vi "simflight-2.0.vi"() -> ()   [LabVIEW 2014]
uses:
  state space loop data.ctl
  <vilib>/addons/Control Design/_Model Construction/Data Typedefs.llb/CD MIMO Time Response Data.ctl
  <vilib>/addons/Control Design/_Model Construction/Data Typedefs.llb/CD Plot Types Enum.ctl
  <vilib>/Utility/miscctls.llb/LV3DPointTypeDef.ctl
  <vilib>/Analysis/baseanly.llb/Real Outer Product.vi
  Data Xfer/subvis/Curcular Buffer Data History.vi
  <vilib>/Analysis/Matrix/Numeric/Subtract/Subtract - RM,RM.vi
  <vilib>/addons/Control Design/_Model Construction/Model Creation.llb/Model Creation SubVI/cd_Create State Space Model.vi
  <vilib>/Utility/inputDevices.llb/joystickAcquire.vi
  <vilib>/addons/Control Design/_Time Response Analysis/Time Response.llb/Time Response subVI/cd_Linear Simulation (State-Space).vi
  <vilib>/addons/Control Design/_Model Construction/NI_LinSys_Model Creation.lvlib
  <vilib>/addons/Control Design/_Time Response Analysis/NI_CD_Time Response.lvlib
  <vilib>/addons/Control Design/_Model Construction/NI_LinSys_Data Typedefs.lvlib
  attitude indicator/lv-attitudecontrol.lvlib
  <vilib>/Analysis/NI_AALBase.lvlib
  <vilib>/Analysis/Matrix/NI_Matrix.lvlib
panel:
  out "altitude 3":T1(graph)
  out "altitude 2":T1(graph)
  out "altitude":T1(graph)
  in  "elevator gain":dbl
  in  "aileron gain":dbl
  in  "rudder gain":dbl
  out "plot":T1(graph)
  in  "Aircraft":string="MPX5"
  in  "Attitude Indicator":refnum<vi>(3d-picture)
  out "Airspeed (ft/s)":dbl(knob)=74.91519927978516 scale=0.0..120.0 scale format="%#.4f"
  out "motor (BHP)":dbl(slide) scale=-0.2..0.2
  out "ground track":cluster{"Time Stamp":dbl, "Data Value":dbl}[](graph)
  out "roll":dbl(slide) scale=-90.0..90.0
  out "pitch":dbl(slide) scale=-90.0..90.0
  out "rudder":dbl(slide) scale=-25.0..25.0
  out "aileron":dbl(slide) scale=-25.0..25.0
  out "elevator":dbl(slide) scale=-25.0..25.0
  out "Heading":T2(graph)={"X"=[{"Y"=[21.620706805998168, 20.15124367946963, 12.465582235692763, 7.946576972490323, 11.656565240893995, 3.970903792227472, 5.440366929130449, 13.126028372052978, 19.003880895383112, 16.244982298473555, 16.832767550897515, 24.922937499080067, 24.33515224168201, 19.81289788882929, 13.93504536742159, 21.620706805998168], "Y"=[7.099604990531346, 5.077062500919932, 10.661022401488875, 5.291796067500631, 11.248807654089271, 16.832767550897515, 18.855310035128806, 13.271350139939326, 21.36152008350073, 25.220079209877188, 26.02909620777253, 20.151243679469633, 19.34222668734553, 20.773734831883043, 12.683564887248515, 7.099604990531346]}], "z"=[{"Y"=[15.0, 16.30733614, 17.60472267, 17.43107449, 17.60472267, 18.88228568, 20.13030215, 19.78828201, 20.13030215, 21.33927393, 22.5, 22.0, 22.5, 23.60364655, 24.64181415, 23.99902654, 24.64181415, 25.60660172, 26.49066665, 25.7246222, 26.49066665, 27.28728066, 27.99038106, 27.12435565, 27.99038106, 28.59461681, 29.09538931, 28.15569669, 29.09538931, 29.48888739, 29.7721163, 28.78730854, 29.7721163, 29.94292047, 30.0, 28.5, 30.0, 29.94292047, 29.7721163, 28.78730854, 29.7721163, 29.48888739, 29.09538931, 28.15569669, 29.09538931, 28.59461681, 27.99038106, 27.12435565, 27.99038106, 27.28728066, 26.49066665, 25.7246222, 26.49066665, 25.60660172, 24.64181415, 23.99902654, 24.64181415, 23.60364655, 22.5, 22.0, 22.5, 21.33927393, 20.13030215, 19.78828201, 20.13030215, 18.88228568, 17.60472267, 17.43107449, 17.60472267, 16.30733614, 15.0, 15.0, 15.0, 13.69266386, 12.39527733, 12.56892551, 12.39527733, 11.11771432, 9.86969785, 10.21171799, 9.86969785, 8.660726074, 7.5, 8.0, 7.5, 6.396353455, 5.358185855, 6.000973464, 5.358185855, 4.393398282, 3.509333353, 4.275377796, 3.509333353, 2.712719336, 2.009618943, 2.875644347, 2.009618943, 1.405383194, 0.904610688, 1.844303309, 0.904610688, 0.511112606, 0.227883705, 1.212691458, 0.227883705, 0.057079529, 0.0, 1.5, 0.0, 0.057079529, 0.227883705, 1.212691458, 0.227883705, 0.511112606, 0.904610688, 1.844303309, 0.904610688, 1.405383194, 2.009618943, 2.875644347, 2.009618943, 2.712719336, 3.509333353, 4.275377796, 3.509333353, 4.393398282, 5.358185855, 6.000973464, 5.358185855, 6.396353455, 7.5, 8.0, 7.5, 8.660726074, 9.86969785, 10.21171799, 9.86969785, 11.11771432, 12.39527733, 12.56892551, 12.39527733, 13.69266386, 15.0, 15.0], "Y"=[30.0, 29.94292047, 29.7721163, 28.78730854, 29.7721163, 29.48888739, 29.09538931, 28.15569669, 29.09538931, 28.59461681, 27.99038106, 27.12435565, 27.99038106, 27.28728066, 26.49066665, 25.7246222, 26.49066665, 25.60660172, 24.64181415, 23.99902654, 24.64181415, 23.60364655, 22.5, 22.0, 22.5, 21.33927393, 20.13030215, 19.78828201, 20.13030215, 18.88228568, 17.60472267, 17.43107449, 17.60472267, 16.30733614, 15.0, 15.0, 15.0, 13.69266386, 12.39527733, 12.56892551, 12.39527733, 11.11771432, 9.86969785, 10.21171799, 9.86969785, 8.660726074, 7.5, 8.0, 7.5, 6.396353455, 5.358185855, 6.000973464, 5.358185855, 4.393398282, 3.509333353, 4.275377796, 3.509333353, 2.712719336, 2.009618943, 2.875644347, 2.009618943, 1.405383194, 0.904610688, 1.844303309, 0.904610688, 0.511112606, 0.227883705, 1.212691458, 0.227883705, 0.057079529, 0.0, 1.5, 0.0, 0.057079529, 0.227883705, 1.212691458, 0.227883705, 0.511112606, 0.904610688, 1.844303309, 0.904610688, 1.405383194, 2.009618943, 2.875644347, 2.009618943, 2.712719336, 3.509333353, 4.275377796, 3.509333353, 4.393398282, 5.358185855, 6.000973464, 5.358185855, 6.396353455, 7.5, 8.0, 7.5, 8.660726074, 9.86969785, 10.21171799, 9.86969785, 11.11771432, 12.39527733, 12.56892551, 12.39527733, 13.69266386, 15.0, 15.0, 15.0, 16.30733614, 17.60472267, 17.43107449, 17.60472267, 18.88228568, 20.13030215, 19.78828201, 20.13030215, 21.33927393, 22.5, 22.0, 22.5, 23.60364655, 24.64181415, 23.99902654, 24.64181415, 25.60660172, 26.49066665, 25.7246222, 26.49066665, 27.28728066, 27.99038106, 27.12435565, 27.99038106, 28.59461681, 29.09538931, 28.15569669, 29.09538931, 29.48888739, 29.7721163, 28.78730854, 29.7721163, 29.94292047, 30.0, 28.5]}]}
  in  "visual":refnum<k7>(container) caption="3D 파라미터형 표면"
  in  "stop":bool
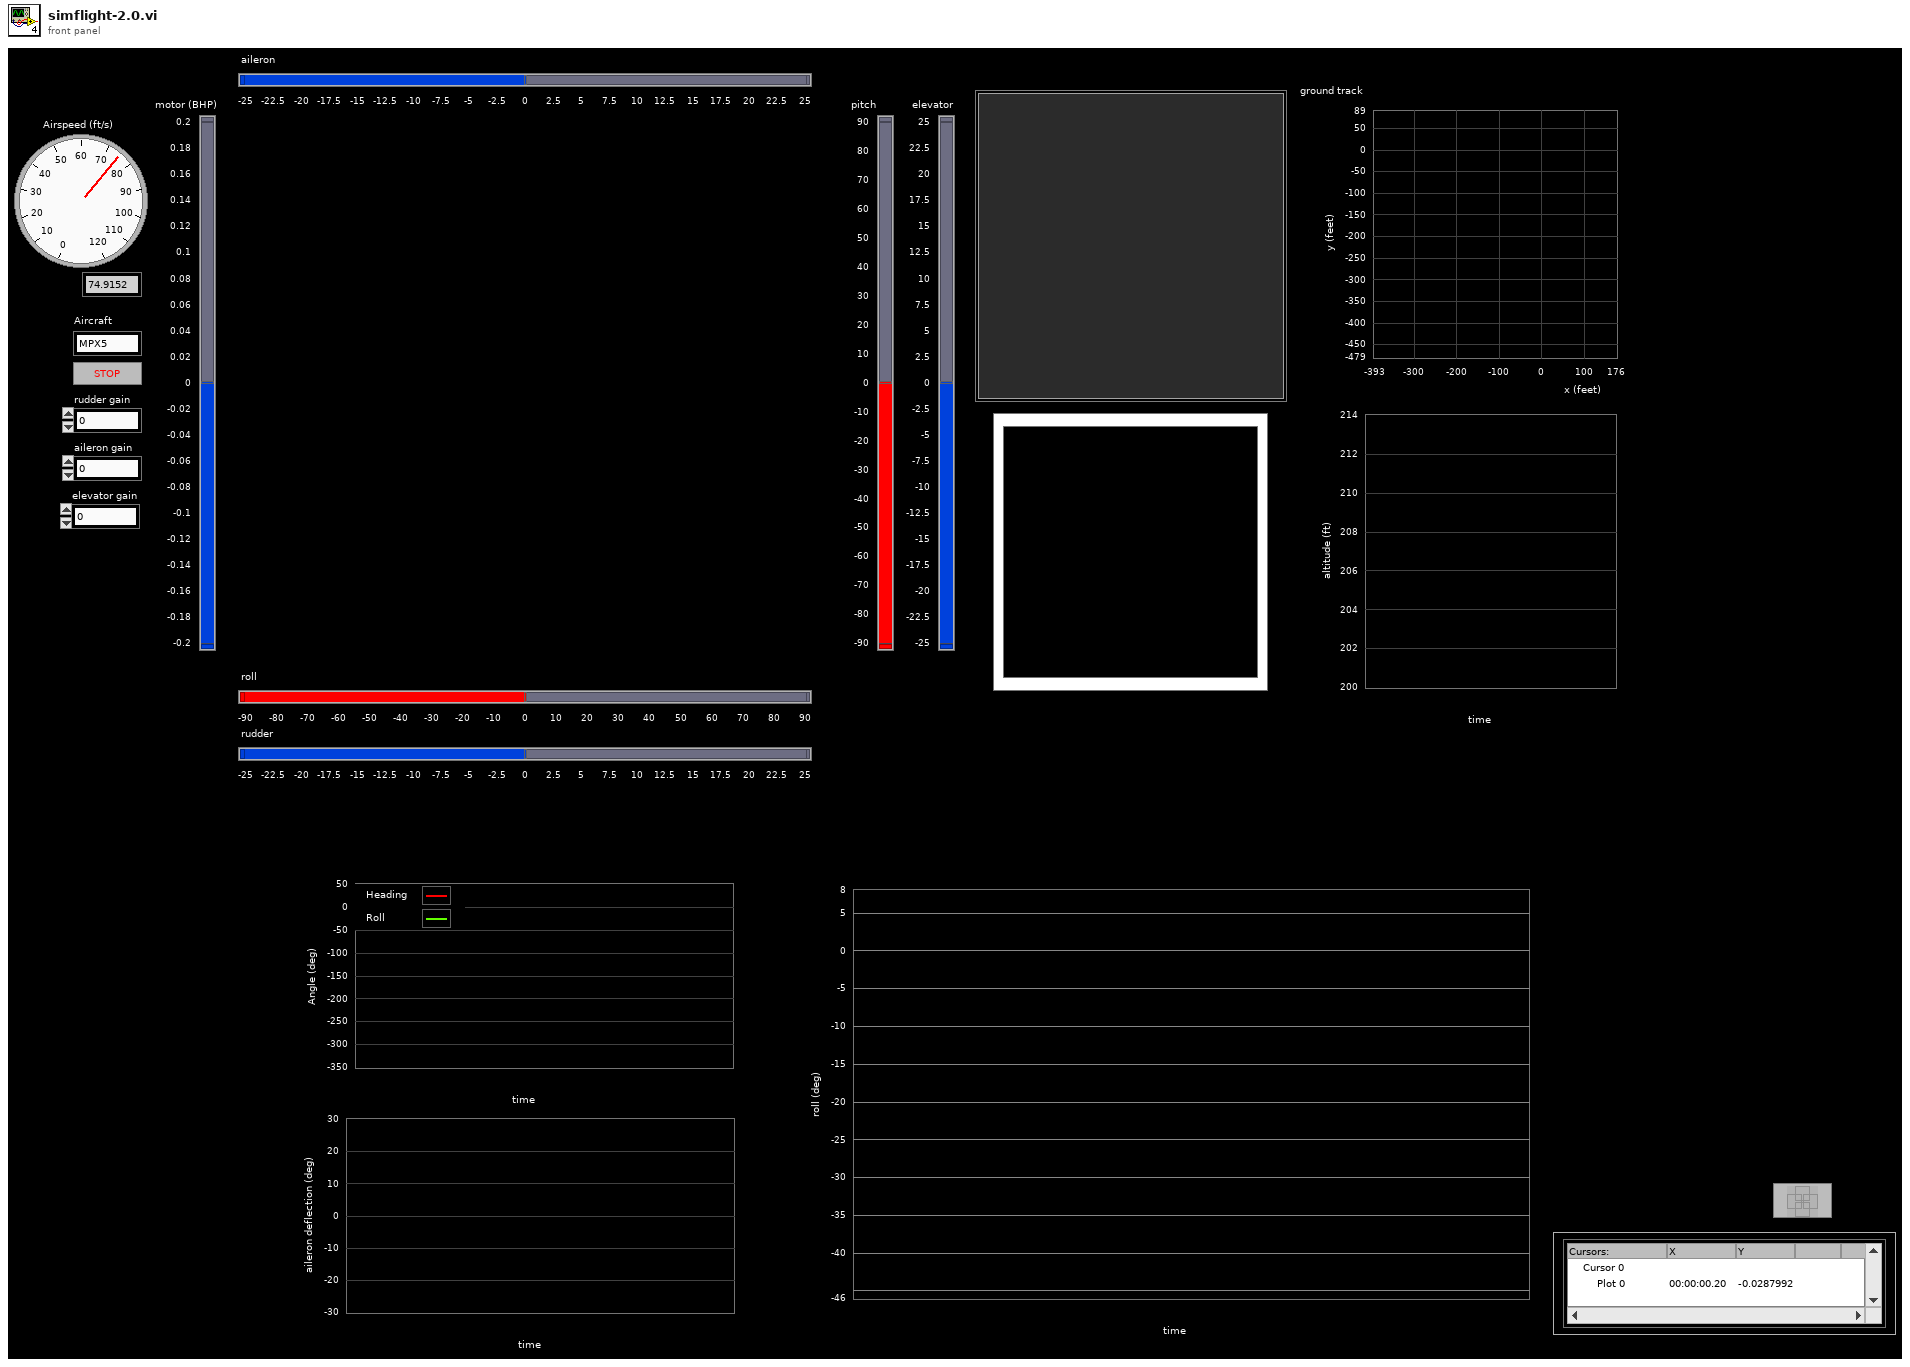
[diagram p1: front panel]
types:
  T1 = cluster{cluster{"Time Stamp":dbl, "Data Value":dbl}[]}[]
  T2 = cluster{"X":cluster{"Y":dbl[], "Y":dbl[]}[], "z":cluster{"Y":dbl[], "Y":dbl[]}[]}
  T3 = typedef "state space loop data.ctl" = cluster{"d_elevator (rad)":dbl, "d_rudder (rad)":dbl, "d_aileron (rad)":dbl, "d_motor (bhp)":dbl, "loop start (s)":dbl, "dT":dbl, "time now":dbl, "Sim Data":T4, "sim conditions":dbl[], "timestamp":dbl}
  T4 = typedef "NI_LinSys_Data Typedefs.lvlib/CD MIMO Time Response Data.ctl" = cluster{"Time":dbl[], "Outputs Data":dbl[][][], "States Data":dbl[][][], "plot type":T5}
  T5 = typedef "NI_LinSys_Data Typedefs.lvlib/CD Plot Types Enum.ctl" = enum16{"bode-magnitude", "bode-phase", "nichols", "nyquist", "singular values", "step", "impulse", "initial", "simulation", "nyquist with separation"}
  T6 = typedef "NI_Matrix.lvlib/RealMatrix.ctl" = dbl[][]
  T7 = typedef "NI_LinSys_Model Typedefs.lvlib/CD State Space Model (MIMO).ctl" = cluster{"properties":T8, "A":dbl[][], "B":dbl[][], "C":dbl[][], "D":dbl[][], "StateNames":string[], "Transport Delay":dbl[][]}
  T8 = typedef "NI_LinSys_Model Typedefs.lvlib/CD General Elements.ctl" = cluster{"Model name":string, "Input names":string[], "Output names":string[], "Input Delays":dbl[], "Output Delays":dbl[], "Sampling Time":dbl, "Notes":string}
  T9 = typedef "lv-attitudecontrol.lvlib/AttitudeHandle.ctl" = cluster{"First Scene Object":refnum<vi>, "Drum":refnum<vi>, "Window":refnum<vi>, "Dial":refnum<vi>, "Scene Graph":refnum<vi>, "Last Drum Pitch":dbl, "Last Drum Roll ":dbl, "Last Dial Roll":dbl}
  T10 = cluster{"X axis":i32, "Y axis":i32, "Z axis":i32, "X axis rotation":i32, "Y axis rotation":i32, "Z axis rotation":i32, "U axis":i32, "V axis":i32}
  T11 = typedef "LV3DPointTypeDef.ctl" = cluster{"X":sgl, "Y":sgl, "Z":sgl}
  T12 = cluster{cluster{"Time Stamp":dbl, "Data Value":dbl}[]}
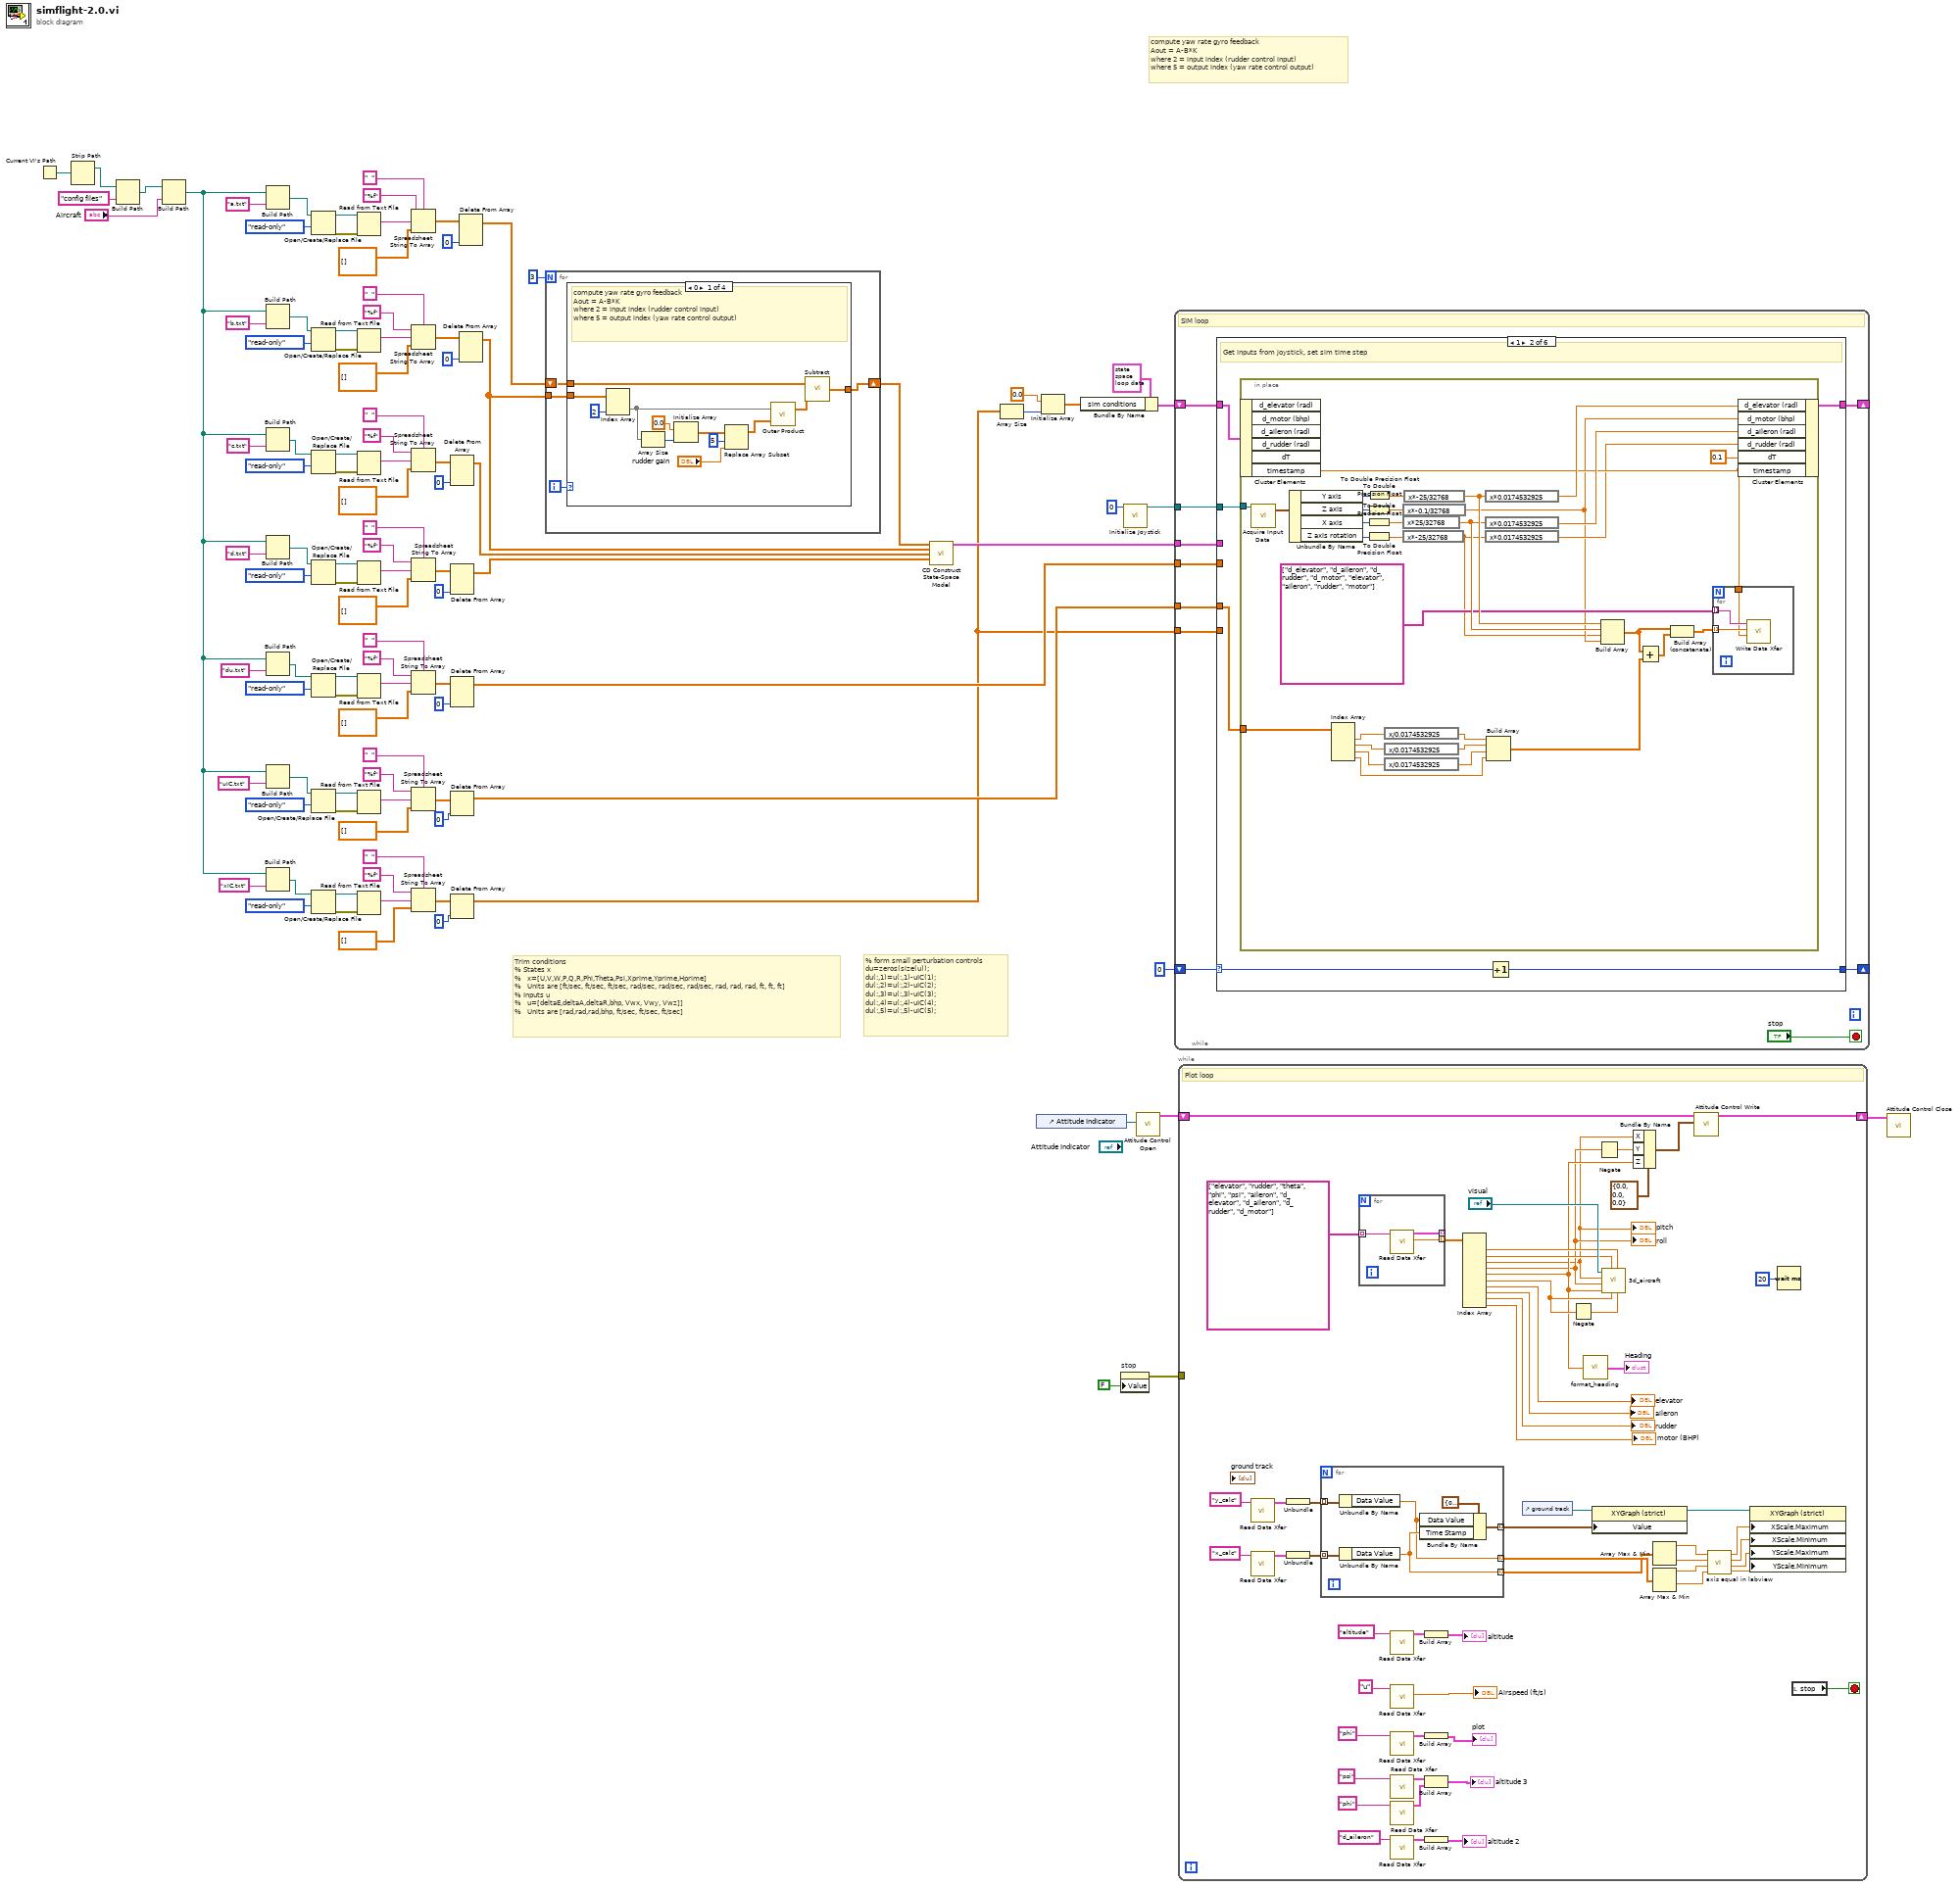
[diagram p0: block diagram]
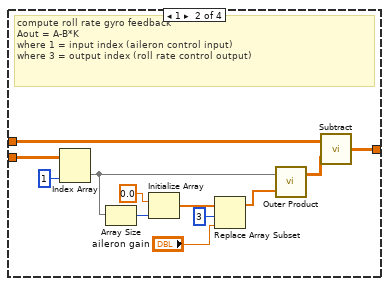
[diagram p2: hidden frame]
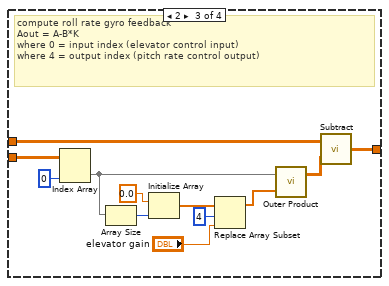
[diagram p3: hidden frame]
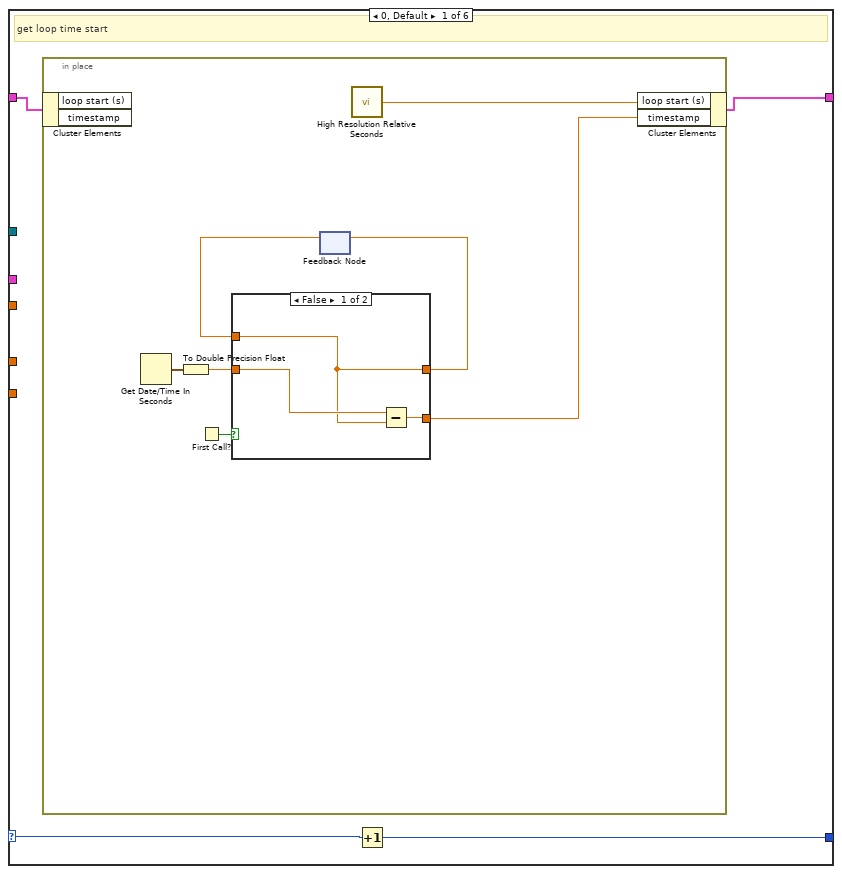
[diagram p5: hidden frame]
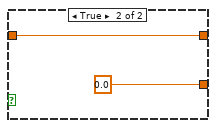
[diagram p6: hidden frame]
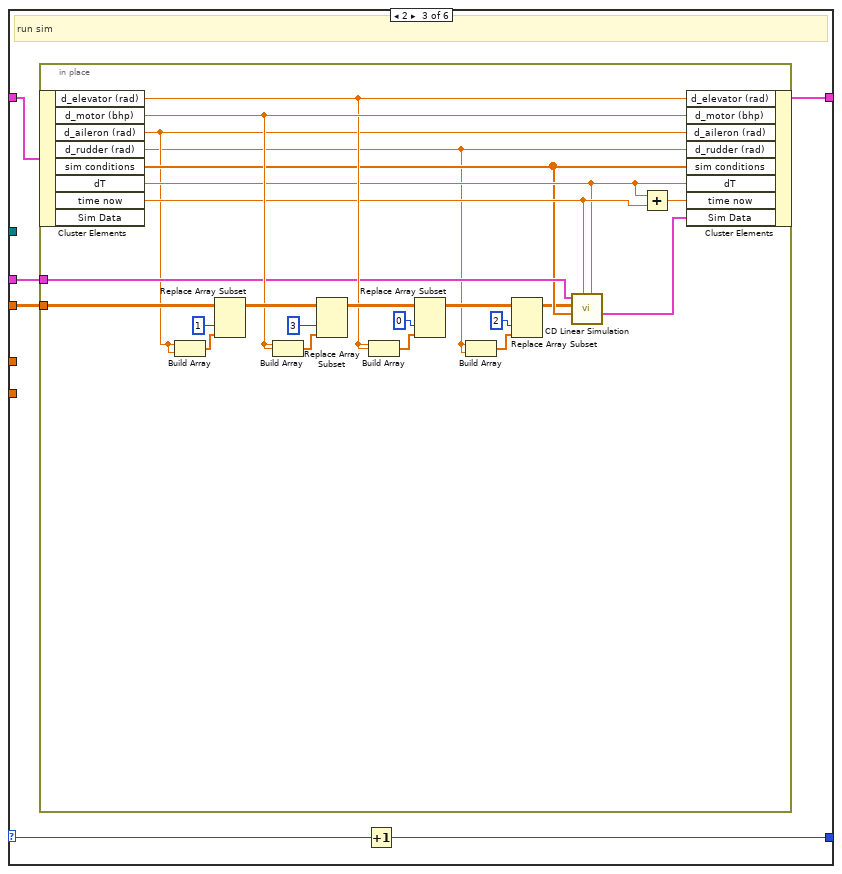
[diagram p7: hidden frame]
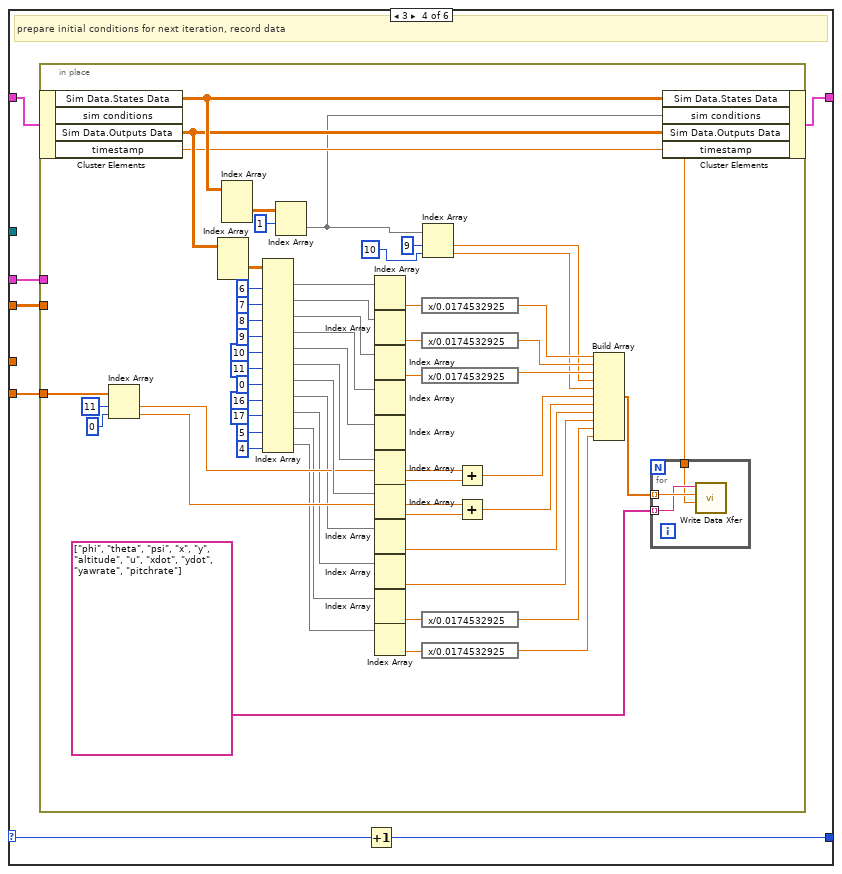
[diagram p8: hidden frame]
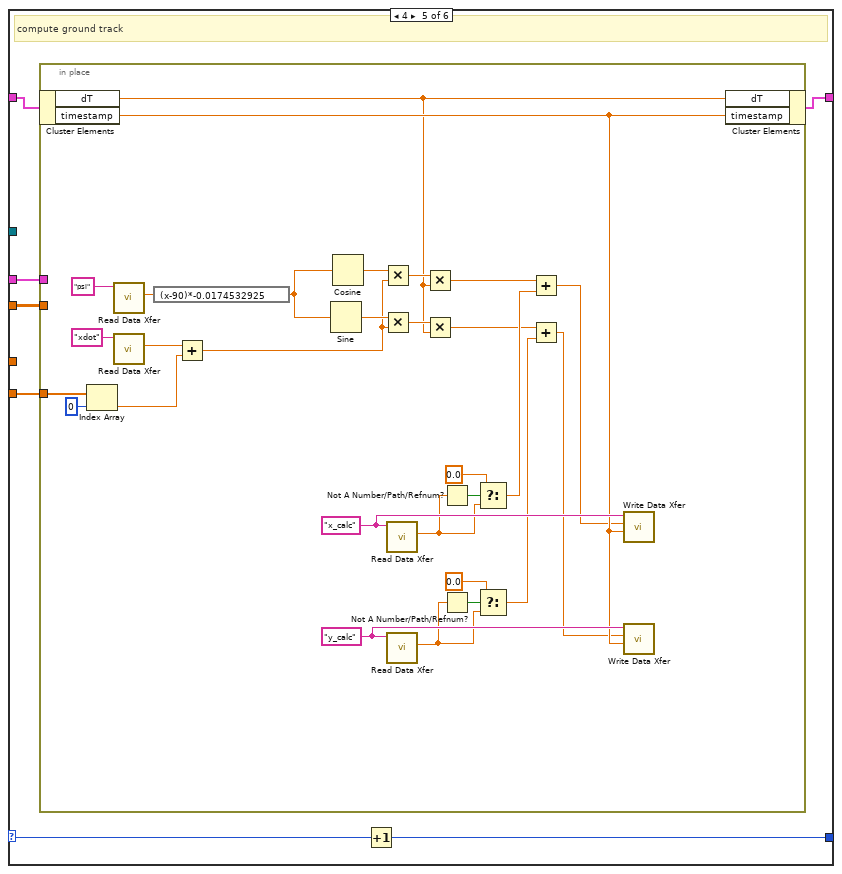
[diagram p9: hidden frame]
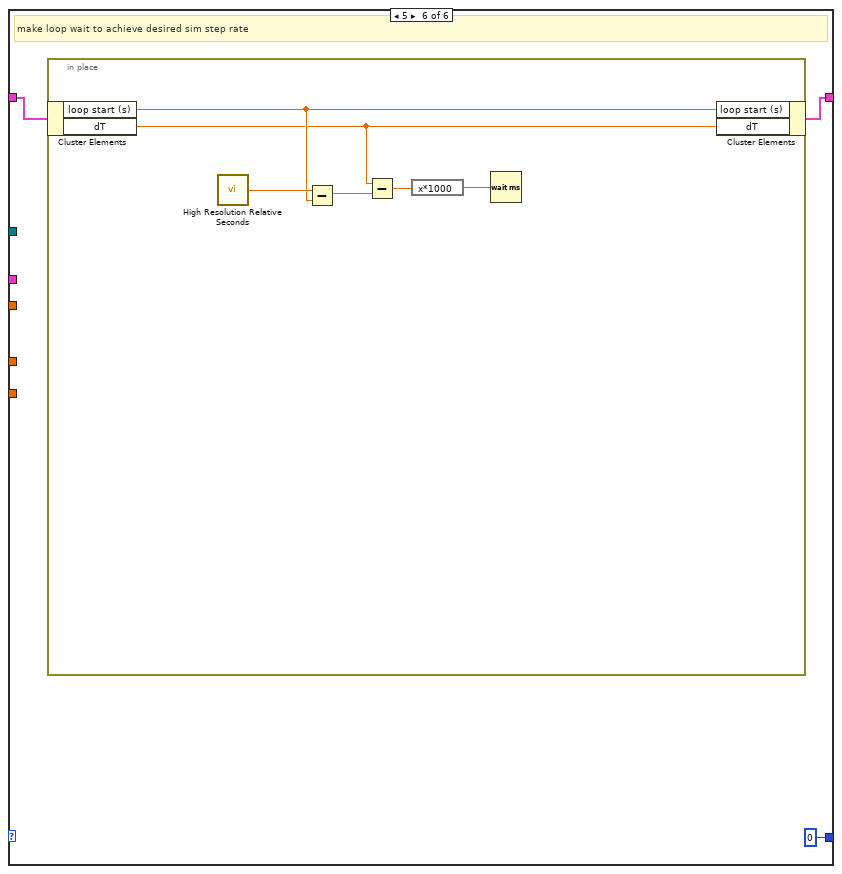
[diagram p10: hidden frame]
diagram:
  # "compute yaw rate gyro feedback\nAout = A-B*K\nwhere 2 = input index (rudder control input)\nwhere 5 = output index (yaw rate control output)"
  # "% form small perturbation controls\ndu=zeros(size(u));\ndu(:,1)=u(:,1)-uIC(1);\ndu(:,2)=u(:,2)-uIC(2);\ndu(:,3)=u(:,3)-uIC(3);\ndu(:,4)=u(:,4)-uIC(4);\ndu(:,5)=u(:,5)-uIC(5);"
  # "Trim conditions\n% States x\n%   x=[U,V,W,P,Q,R,Phi,Theta,Psi,Xprime,Yprime,Hprime]\n%   Units are [ft/sec, ft/sec, ft/sec, rad/sec, rad/sec, rad/sec, rad, rad, rad, ft, ft, ft]\n% Inputs u\n%   u=[deltaE,deltaA,deltaR,bhp, Vwx, Vwy, Vwz]]\n%   Units are [rad,rad,rad,bhp, ft/sec, ft/sec, ft/sec]"
  n1 = Current VI's Path() -> (path=w34:path)
  n2 = Strip Path(path=w34) -> (stripped path=w33:path)  [unwired: 1 out]
  n3 = Build Path(base path=w33, name or relative path="config files") -> (appended path=w50:path)
  n4 = Build Path(base path=w50, name or relative path="Aircraft") -> (appended path=w32:path)
  n5 = Build Path(base path=w32, name or relative path="a.txt") -> (appended path=w47:path)
  n6 = Build Path(base path=w32, name or relative path="b.txt") -> (appended path=w45:path)
  n7 = Build Path(base path=w32, name or relative path="c.txt") -> (appended path=w43:path)
  n8 = Build Path(base path=w32, name or relative path="d.txt") -> (appended path=w41:path)
  n9 = Build Path(base path=w32, name or relative path="du.txt") -> (appended path=w39:path)
  n10 = Build Path(base path=w32, name or relative path="uIC.txt") -> (appended path=w37:path)
  n11 = Build Path(base path=w32, name or relative path="xIC.txt") -> (appended path=w35:path)
  n12 = Open/Create/Replace File(file path (use dialog)=w47, access (0:read/write)=enum16{"read/write", "read-only", "write-only"}."read-only") -> (refnum out=w104:refnum<file>, error out=w105:errorcluster)  [unwired: 4 in, 1 out]
  n13 = Open/Create/Replace File(file path (use dialog)=w45, access (0:read/write)=enum16{"read/write", "read-only", "write-only"}."read-only") -> (refnum out=w97:refnum<file>, error out=w96:errorcluster)  [unwired: 4 in, 1 out]
  n14 = Open/Create/Replace File(file path (use dialog)=w43, access (0:read/write)=enum16{"read/write", "read-only", "write-only"}."read-only") -> (refnum out=w92:refnum<file>, error out=w93:errorcluster)  [unwired: 4 in, 1 out]
  n15 = Open/Create/Replace File(file path (use dialog)=w41, access (0:read/write)=enum16{"read/write", "read-only", "write-only"}."read-only") -> (refnum out=w85:refnum<file>, error out=w84:errorcluster)  [unwired: 4 in, 1 out]
  n16 = Open/Create/Replace File(file path (use dialog)=w39, access (0:read/write)=enum16{"read/write", "read-only", "write-only"}."read-only") -> (refnum out=w80:refnum<file>, error out=w81:errorcluster)  [unwired: 4 in, 1 out]
  n17 = Open/Create/Replace File(file path (use dialog)=w37, access (0:read/write)=enum16{"read/write", "read-only", "write-only"}."read-only") -> (refnum out=w63:refnum<file>, error out=w64:errorcluster)  [unwired: 4 in, 1 out]
  n18 = Open/Create/Replace File(file path (use dialog)=w35, access (0:read/write)=enum16{"read/write", "read-only", "write-only"}."read-only") -> (refnum out=w74:refnum<file>, error out=w75:errorcluster)  [unwired: 4 in, 1 out]
  n19 = Read from Text File(file (use dialog)=w104, error in=w105) -> (text=w103:string)  [unwired: 2 in, 3 out]
  n20 = Read from Text File(file (use dialog)=w97, error in=w96) -> (text=w98:string)  [unwired: 2 in, 3 out]
  n21 = Read from Text File(file (use dialog)=w92, error in=w93) -> (text=w91:string)  [unwired: 2 in, 3 out]
  n22 = Read from Text File(file (use dialog)=w85, error in=w84) -> (text=w86:string)  [unwired: 2 in, 3 out]
  n23 = Read from Text File(file (use dialog)=w80, error in=w81) -> (text=w79:string)  [unwired: 2 in, 3 out]
  n24 = Read from Text File(file (use dialog)=w63, error in=w64) -> (text=w62:string)  [unwired: 2 in, 3 out]
  n25 = Read from Text File(file (use dialog)=w74, error in=w75) -> (text=w73:string)  [unwired: 2 in, 3 out]
  n26 = Spreadsheet String To Array(delimiter (Tab)="  ", format string="%f", spreadsheet string=w103, array type (2D Dbl)=dbl[][] []) -> (array=w20:dbl[][])
  n27 = Spreadsheet String To Array(delimiter (Tab)="  ", format string="%f", spreadsheet string=w98, array type (2D Dbl)=dbl[][] []) -> (array=w17:dbl[][])
  n28 = Spreadsheet String To Array(delimiter (Tab)="  ", format string="%f", spreadsheet string=w91, array type (2D Dbl)=dbl[][] []) -> (array=w14:dbl[][])
  n29 = Spreadsheet String To Array(delimiter (Tab)="  ", format string="%f", spreadsheet string=w86, array type (2D Dbl)=dbl[][] []) -> (array=w11:dbl[][])
  n30 = Spreadsheet String To Array(delimiter (Tab)="  ", format string="%f", spreadsheet string=w79, array type (2D Dbl)=dbl[][] []) -> (array=w8:dbl[][])
  n31 = Spreadsheet String To Array(delimiter (Tab)="  ", format string="%f", spreadsheet string=w62, array type (2D Dbl)=dbl[] []) -> (array=w6:dbl[])
  n32 = Spreadsheet String To Array(delimiter (Tab)="  ", format string="%f", spreadsheet string=w73, array type (2D Dbl)=dbl[] []) -> (array=w2:dbl[])
  n33 = Delete From Array(array=w14, index (col)=0 ("disabled index (col)")) -> (array with subset deleted=w13:dbl[][])  [unwired: 2 in, 1 out]
  n34 = Delete From Array(array=w11, index (col)=0 ("disabled index (col)")) -> (array with subset deleted=w10:dbl[][])  [unwired: 2 in, 1 out]
  n35 = Delete From Array(array=w8, index (col)=0 ("disabled index (col)")) -> (array with subset deleted=w7:dbl[][])  [unwired: 2 in, 1 out]
  n36 = Delete From Array(array=w6, index=0 ("disabled index (col)")) -> (array with subset deleted=w4:dbl[])  [unwired: 1 in, 1 out]
  n37 = Delete From Array(array=w2, index=0 ("disabled index (col)")) -> (array with subset deleted=w1:dbl[])  [unwired: 1 in, 1 out]
  n38 = Delete From Array(array=w20, index (col)=0 ("disabled index (col)")) -> (array with subset deleted=w19:dbl[][])  [unwired: 2 in, 1 out]
  n39 = Delete From Array(array=w17, index (col)=0 ("disabled index (col)")) -> (array with subset deleted=w16:dbl[][])  [unwired: 2 in, 1 out]
  n40 = for {
    N: 3 -> [_]
    tunnel: w16 -> [w110]
    shift-right: [w108] -> w31
    shift-left: w19 -> [w109]
    i -> [w107]
    n41 = case shown="0" w107 {
      tunnel: w110 -> [w122 w134 w146 _]
      tunnel: w109 -> [w121 w133 w145 w147]
      tunnel: [w120 w132 w144 w147] -> w108
      frame 0 {
        # "compute yaw rate gyro feedback\nAout = A-B*K\nwhere 2 = input index (rudder control input)\nwhere 5 = output index (yaw rate control output)"
        n42 = Index Array(array=w122, index (col)=2 ("disabled index (col)")) -> (element=w115:dbl[])  [unwired: 1 in]
        n43 = Array Size(array=w115) -> (size(s)=w116:i32)
        n44 = Initialize Array(0.0, w116) -> (w114:dbl[])
        n45 = Replace Array Subset(array=w114, new element="rudder gain", index=5) -> (w111:dbl[])
        n46 = call-poly <vilib>:"Outer Product.vi"("Y Vector"=w111, "X Vector"=w115) -> ("Outer Product"=w118:T6)  [unwired: 1 out]
        n47 = call-poly <vilib>:"Subtract.vi"("Real Matrix B"=w118, "Real Matrix A"=w121) -> ("A - B"=w120:T6)
      }
      frame 1 {
        # "compute roll rate gyro feedback\nAout = A-B*K\nwhere 1 = input index (aileron control input)\nwhere 3 = output index (roll rate control output)"
        n48 = Index Array(array=w134, index (col)=1 ("disabled index (col)")) -> (element=w127:dbl[])  [unwired: 1 in]
        n49 = Array Size(array=w127) -> (size(s)=w128:i32)
        n50 = Initialize Array(0.0, w128) -> (w126:dbl[])
        n51 = Replace Array Subset(array=w126, new element="aileron gain", index=3) -> (w123:dbl[])
        n52 = call-poly <vilib>:"Outer Product.vi"("Y Vector"=w123, "X Vector"=w127) -> ("Outer Product"=w130:T6)  [unwired: 1 out]
        n53 = call-poly <vilib>:"Subtract.vi"("Real Matrix B"=w130, "Real Matrix A"=w133) -> ("A - B"=w132:T6)
      }
      frame 2 {
        # "compute roll rate gyro feedback\nAout = A-B*K\nwhere 0 = input index (elevator control input)\nwhere 4 = output index (pitch rate control output)"
        n54 = Index Array(array=w146, index (col)=0 ("disabled index (col)")) -> (element=w139:dbl[])  [unwired: 1 in]
        n55 = Array Size(array=w139) -> (size(s)=w140:i32)
        n56 = Initialize Array(0.0, w140) -> (w138:dbl[])
        n57 = Replace Array Subset(array=w138, new element="elevator gain", index=4) -> (w135:dbl[])
        n58 = call-poly <vilib>:"Outer Product.vi"("Y Vector"=w135, "X Vector"=w139) -> ("Outer Product"=w142:T6)  [unwired: 1 out]
        n59 = call-poly <vilib>:"Subtract.vi"("Real Matrix B"=w142, "Real Matrix A"=w145) -> ("A - B"=w144:T6)
      }
      frame Default {
        # "not used"
      }
    }
  }
  n60 = call-poly <vilib>:"CD Construct State-Space Model.vi"("A"=w31, "B"=w16, "C"=w13, "D"=w10) -> ("State-Space Model"=w29:T7)  [unwired: 10 in, 1 out]
  n61 = Array Size(array=w1) -> (size(s)=w57:i32)
  n62 = control-ref of="Attitude Indicator"() -> (w54:refnum<vi>)
  n63 = Initialize Array(0.0, w57) -> (w55:dbl[])
  n64 = Bundle By Name(cluster=T3 {"d_elevator (rad)"=0.0, "d_rudder (rad)"=0.0, "d_aileron (rad)"=0.0, "d_motor (bhp)"=0.0, "loop start (s)"=0.0, "dT"=0.0, "time now"=0.0, "Sim Data"={"Time"=[], "Outputs Data"=[], "States Data"=[], "plot type"=enum."step"}, "sim conditions"=[], "timestamp"=0.0}, "sim conditions"=w55) -> (w66:T3)
  n65 = property on="stop" class="Bool (strict)"("Value"=FALSE ("stop")) -> (error out=w58:errorcluster)  [unwired: 2 in, 1 out]
  n66 = call <vilib>:"Initialize Joystick.vi"("device index"=0) -> ("device ID"=w69:refnum<k1>)  [unwired: 9 in, 1 out]
  n67 = call "Attitude Control Open.vi"("Scene Graph"=w54) -> ("Attitude Control Handle"=w53:T9)  [unwired: 9 in, 1 out]
  n68 = while {
    shift-right: [w156] -> _
    shift-left: w66 -> [w157]
    tunnel: w69 -> [w155]
    shift-right: [w154] -> _
    shift-left: 0 -> [w153]
    tunnel: w29 -> [w151]
    tunnel: w7 -> [w150]
    tunnel: w4 -> [w149]
    tunnel: w1 -> [w148]
    stop <- "stop" stop-if-true
    # "SIM loop"
    n69 = case shown="1" w153 {
      tunnel: w157 -> [w159 w178 w220 w250 w316 w347]
      tunnel: [w158 w177 w219 w249 w315 w346] -> w156
      tunnel: w155 -> [_ w179 _ _ _ _]
      selector: w153 -> [w161 w176 w218 w248 w314 _]
      tunnel: [w160 w175 w217 w247 w313 0] -> w154
      tunnel: w151 -> [_ _ w215 w245 w311 _]
      tunnel: w150 -> [_ _ w216 w246 w312 _]
      tunnel: w149 -> [_ w174 _ _ _ _]
      tunnel: w148 -> [_ _ _ w244 w310 _]
      frame 0, Default {
        # "get loop time start"
        n70 = in-place {
          n71 = in-place-cluster #1(w159) -> ()  [unwired: 2 out]
          n72 = Get Date/Time In Seconds() -> (seconds since 1Jan1904=w167:timestamp)
          n73 = To Double Precision Float(number=w167) -> (double precision float=w165:dbl)
          n74 = First Call?() -> (First Call?: T/F=w166:bool)
          n75 = feedback #2() -> (w163:dbl)  [unwired: 1 in]
          n76 = case shown="False" w166 {
            tunnel: w165 -> [w170 w173]
            tunnel: [w169 w173] -> w164
            tunnel: w163 -> [w169 _]
            tunnel: [w171 0.0] -> w162
            frame False {
              n77 = Subtract(x=w170, y=w169) -> (x-y=w171:dbl)
            }
            frame True {
            }
          }
          n78 = feedback-in #2(w164) -> ()
          n79 = call <vilib>:"High Resolution Relative Seconds.vi"() -> ("relative seconds"=w168:dbl)
          n80 = in-place-cluster #1("loop start (s)"=w168, "timestamp"=w162) -> (w158:T3)
        }
        n81 = Increment(x=w161) -> (x+1=w160:i32)
      }
      frame 1 {
        # "Get inputs from joystick, set sim time step"
        n82 = in-place {
          in-place-border: w179 -> [w209]
          in-place-border: w174 -> [w197]
          n83 = in-place-cluster #3(w178) -> ("timestamp"=w198:dbl)  [unwired: 5 out]
          n84 = call-poly <vilib>:"Acquire Input Data.vi"("device ID"=w209) -> ("axis info"=w208:T10)  [unwired: 14 in, 4 out]
          n85 = Unbundle By Name(w208) -> ("Y axis"=w210:i32, "Z axis"=w205:i32, "X axis"=w204:i32, "Z axis rotation"=w187:i32)
          n86 = Index Array(array=w197) -> (element #1=w192:dbl, element #2=w190:dbl, element #3=w182:dbl, element #4=w180:dbl)  [unwired: 4 in]
          n87 = To Double Precision Float(number=w205) -> (double precision float=w206:dbl)
          n88 = To Double Precision Float(number=w204) -> (double precision float=w188:dbl)
          n89 = To Double Precision Float(number=w187) -> (double precision float=w186:dbl)
          n90 = To Double Precision Float(number=w210) -> (double precision float=w211:dbl)
          n91 = expression code="x/0.0174532925"(w192) -> (w191:dbl)
          n92 = expression code="x/0.0174532925"(w190) -> (w189:dbl)
          n93 = expression code="x/0.0174532925"(w182) -> (w181:dbl)
          n94 = expression code="x*-0.1/32768"(w206) -> (w184:dbl)
          n95 = expression code="x*25/32768"(w188) -> (w200:dbl)
          n96 = expression code="x*-25/32768"(w186) -> (w183:dbl)
          n97 = expression code="x*-25/32768"(w211) -> (w201:dbl)
          n98 = expression code="x*0.0174532925"(w201) -> (w207:dbl)
          n99 = expression code="x*0.0174532925"(w200) -> (w203:dbl)
          n100 = expression code="x*0.0174532925"(w183) -> (w185:dbl)
          n101 = Build Array(w191, w189, w181, w180) -> (w196:dbl[])
          n102 = Build Array(w201, w200, w183, w184) -> (w194:dbl[])
          n103 = Add(x=w194, y=w196) -> (x+y=w195:dbl[])
          n104 = Build Array (concatenate)(w194, w195) -> (w193:dbl[])
          n105 = for {
            tunnel: w193 -> [w214] mode=indexing
            tunnel: string[] ["d_elevator", "d_aileron", "d_rudder", "d_motor", "elevator", "aileron", "rudder", "motor"] -> [w213] mode=indexing
            tunnel: w198 -> [w212]
            n106 = call "Write Data Xfer.vi"("Time Stamp"=w212, "Data Value"=w214, "Device Name"=w213) -> ()  [unwired: 8 in, 1 out]
          }
          n107 = in-place-cluster #3("d_elevator (rad)"=w207, "d_motor (bhp)"=w184, "d_aileron (rad)"=w203, "d_rudder (rad)"=w185, "dT"=0.1, "timestamp"=w198) -> (w177:T3)
        }
        n108 = Increment(x=w176) -> (x+1=w175:i32)
      }
      frame 2 {
        # "run sim"
        n109 = in-place {
          in-place-border: w216 -> [w238]
          in-place-border: w215 -> [w232]
          n110 = in-place-cluster #4(w220) -> ("d_elevator (rad)"=w233:dbl, "d_motor (bhp)"=w235:dbl, "d_aileron (rad)"=w226:dbl, "d_rudder (rad)"=w221:dbl, "sim conditions"=w227:dbl[], "dT"=w230:dbl, "time now"=w231:dbl)  [unwired: 1 out]
          n111 = Build Array(w226, w226) -> (w237:dbl[])
          n112 = Replace Array Subset(array=w238, new element=w237, index (col)=1 ("disabled index (col)")) -> (w243:dbl[][])  [unwired: 1 in]
          n113 = Build Array(w235, w235) -> (w236:dbl[])
          n114 = Replace Array Subset(array=w243, new element=w236, index (col)=3 ("disabled index (col)")) -> (w240:dbl[][])  [unwired: 1 in]
          n115 = Build Array(w233, w233) -> (w234:dbl[])
          n116 = Replace Array Subset(array=w240, new element=w234, index (col)=0 ("index")) -> (w223:dbl[][])  [unwired: 1 in]
          n117 = Build Array(w221, w221) -> (w225:dbl[])
          n118 = Replace Array Subset(array=w223, new element=w225, index (col)=2 ("index")) -> (w222:dbl[][])  [unwired: 1 in]
          n119 = call-poly <vilib>:"CD Linear Simulation.vi"("Delta t"=w230, "Initial Time"=w231, "Initial Conditions"=w227, "Inputs"=w222, "State-Space Model"=w232) -> ("Simulation Data"=w228:T4)  [unwired: 3 in, 3 out]
          n120 = Add(x=w230, y=w231) -> (x+y=w229:dbl)
          n121 = in-place-cluster #4("d_elevator (rad)"=w233, "d_motor (bhp)"=w235, "d_aileron (rad)"=w226, "d_rudder (rad)"=w221, "sim conditions"=w227, "dT"=w230, "time now"=w229, "Sim Data"=w228) -> (w219:T3)
        }
        n122 = Increment(x=w218) -> (x+1=w217:i32)
      }
      frame 3 {
        # "prepare initial conditions for next iteration, record data"
        n123 = in-place {
          in-place-border: w246 -> [_]
          in-place-border: w245 -> [_]
          in-place-border: w244 -> [w278]
          n124 = in-place-cluster #5(w250) -> ("Sim Data.States Data"=w304:dbl[][][], "Sim Data.Outputs Data"=w303:dbl[][][], "timestamp"=w286:dbl)  [unwired: 1 out]
          n125 = Index Array(array=w278, index #1=11 ("index"), index #2=0 ("index")) -> (element #1=w276:dbl, element #2=w271:dbl)
          n126 = Index Array(array=w303) -> (element=w302:dbl[][])  [unwired: 3 in]
          n127 = Index Array(array=w304) -> (element=w305:dbl[][])  [unwired: 3 in]
          n128 = Index Array(array=w302, index (col) #1=6 ("disabled index (col)"), index (col) #2=7 ("disabled index (col)"), index (col) #3=8 ("disabled index (col)"), index (col) #4=9 ("disabled index (col)"), index (col) #5=10 ("disabled index (col)"), index (col) #6=11 ("disabled index (col)"), index (col) #7=0 ("disabled index (col)"), index (col) #8=16 ("disabled index (col)"), index (col) #9=17 ("disabled index (col)"), index (col) #10=5 ("disabled index (col)"), index (col) #11=4 ("disabled index (col)")) -> (element #1=w300:dbl[], element #2=w299:dbl[], element #3=w298:dbl[], element #4=w297:dbl[], element #5=w296:dbl[], element #6=w295:dbl[], element #7=w279:dbl[], element #8=w267:dbl[], element #9=w266:dbl[], element #10=w255:dbl[], element #11=w253:dbl[])  [unwired: 11 in]
          n129 = Index Array(array=w305, index (row)=1) -> (element=w263:dbl[])  [unwired: 1 in]
          n130 = Index Array(array=w300) -> (element #2=w294:dbl)  [unwired: 2 in, 1 out]
          n131 = Index Array(array=w299) -> (element #2=w291:dbl)  [unwired: 2 in, 1 out]
          n132 = Index Array(array=w298) -> (element #2=w290:dbl)  [unwired: 2 in, 1 out]
          n133 = Index Array(array=w297) -> ()  [unwired: 2 in, 2 out]
          n134 = Index Array(array=w296) -> ()  [unwired: 2 in, 2 out]
          n135 = Index Array(array=w295) -> (element #2=w277:dbl)  [unwired: 2 in, 1 out]
          n136 = Index Array(array=w279) -> (element #2=w272:dbl)  [unwired: 2 in, 1 out]
          n137 = Index Array(array=w267) -> (element #2=w264:dbl)  [unwired: 2 in, 1 out]
          n138 = Index Array(array=w266) -> (element #2=w265:dbl)  [unwired: 2 in, 1 out]
          n139 = Index Array(array=w255) -> (element #2=w256:dbl)  [unwired: 2 in, 1 out]
          n140 = Index Array(array=w253) -> (element #2=w252:dbl)  [unwired: 2 in, 1 out]
          n141 = expression code="x/0.0174532925"(w294) -> (w285:dbl)
          n142 = expression code="x/0.0174532925"(w291) -> (w284:dbl)
          n143 = expression code="x/0.0174532925"(w290) -> (w283:dbl)
          n144 = expression code="x/0.0174532925"(w256) -> (w257:dbl)
          n145 = expression code="x/0.0174532925"(w252) -> (w251:dbl)
          n146 = Index Array(array=w263, index #1=9 ("index"), index #2=10 ("index")) -> (element #1=w261:dbl, element #2=w260:dbl)
          n147 = Add(x=w276, y=w277) -> (x+y=w273:dbl)
          n148 = Add(x=w271, y=w272) -> (x+y=w270:dbl)
          n149 = Build Array(w285, w284, w283, w261, w260, w273, w270, w264, w265, w257, w251) -> (w282:dbl[])
          n150 = for {
            tunnel: w282 -> [w309] mode=indexing
            tunnel: string[] ["phi", "theta", "psi", "x", "y", "altitude", "u", "xdot", "ydot", "yawrate", "pitchrate"] -> [w308] mode=indexing
            tunnel: w286 -> [w307]
            n151 = call "Write Data Xfer.vi"("Time Stamp"=w307, "Data Value"=w309, "Device Name"=w308) -> ()  [unwired: 8 in, 1 out]
          }
          n152 = in-place-cluster #5("Sim Data.States Data"=w304, "sim conditions"=w263, "Sim Data.Outputs Data"=w303, "timestamp"=w286) -> (w249:T3)
        }
        n153 = Increment(x=w248) -> (x+1=w247:i32)
      }
      frame 4 {
        # "compute ground track"
        n154 = in-place {
          in-place-border: w312 -> [_]
          in-place-border: w311 -> [_]
          in-place-border: w310 -> [w334]
          w343 = "x_calc"
          w344 = "y_calc"
          n155 = in-place-cluster #6(w316) -> ("dT"=w323:dbl, "timestamp"=w342:dbl)
          n156 = Index Array(array=w334, index=0) -> (element=w333:dbl)
          n157 = call "Read Data Xfer.vi"("Device Name"="psi") -> ("Latest Value"=w330:dbl)  [unwired: 7 in, 3 out]
          n158 = call "Read Data Xfer.vi"("Device Name"="xdot") -> ("Latest Value"=w332:dbl)  [unwired: 7 in, 3 out]
          n159 = expression code="(x-90)*-0.0174532925"(w330) -> (w329:dbl)
          n160 = Add(x=w332, y=w333) -> (x+y=w326:dbl)
          n161 = Sine(x=w329) -> (sin(x)=w327:dbl)
          n162 = Cosine(x=w329) -> (cos(x)=w328:dbl)
          n163 = Multiply(x=w328, y=w326) -> (x*y=w325:dbl)
          n164 = Multiply(x=w327, y=w326) -> (x*y=w324:dbl)
          n165 = call "Read Data Xfer.vi"("Device Name"=w343) -> ("Latest Value"=w339:dbl)  [unwired: 7 in, 3 out]
          n166 = call "Read Data Xfer.vi"("Device Name"=w344) -> ("Latest Value"=w336:dbl)  [unwired: 7 in, 3 out]
          n167 = Multiply(x=w325, y=w323) -> (x*y=w322:dbl)
          n168 = Multiply(x=w324, y=w323) -> (x*y=w319:dbl)
          n169 = Not A Number/Path/Refnum?(number/path/refnum=w339) -> (NaN/Path/Refnum?=w341:bool)
          n170 = Not A Number/Path/Refnum?(number/path/refnum=w336) -> (NaN/Path/Refnum?=w337:bool)
          n171 = Select(t=0.0, s=w341, f=w339) -> (s? t:f=w321:dbl)
          n172 = Select(t=0.0, s=w337, f=w336) -> (s? t:f=w318:dbl)
          n173 = Add(x=w322, y=w321) -> (x+y=w320:dbl)
          n174 = Add(x=w319, y=w318) -> (x+y=w317:dbl)
          n175 = call "Write Data Xfer.vi"("Time Stamp"=w342, "Data Value"=w320, "Device Name"=w343) -> ()  [unwired: 8 in, 1 out]
          n176 = call "Write Data Xfer.vi"("Time Stamp"=w342, "Data Value"=w317, "Device Name"=w344) -> ()  [unwired: 8 in, 1 out]
          n177 = in-place-cluster #6("dT"=w323, "timestamp"=w342) -> (w315:T3)
        }
        n178 = Increment(x=w314) -> (x+1=w313:i32)
      }
      frame 5 {
        # "make loop wait to achieve desired sim step rate"
        n179 = in-place {
          n180 = in-place-cluster #7(w347) -> ("loop start (s)"=w352:dbl, "dT"=w351:dbl)
          n181 = call <vilib>:"High Resolution Relative Seconds.vi"() -> ("relative seconds"=w354:dbl)
          n182 = Subtract(x=w354, y=w352) -> (x-y=w353:dbl)
          n183 = Subtract(x=w351, y=w353) -> (x-y=w349:dbl)
          n184 = expression code="x*1000"(w349) -> (w350:dbl)
          n185 = Wait (ms)(milliseconds to wait=w350) -> ()  [unwired: 1 out]
          n186 = in-place-cluster #7("loop start (s)"=w352, "dT"=w351) -> (w346:T3)
        }
      }
    }
  }
  n187 = while {
    tunnel: w58 -> [_]
    shift-right: [w383] -> w52
    shift-left: w53 -> [w385]
    stop <- w411 stop-if-true
    # "Plot loop"
    n188 = call "Read Data Xfer.vi"("Device Name"="y_calc") -> ("Truncated Data History"=w396:T12)  [unwired: 7 in, 3 out]
    n189 = call "Read Data Xfer.vi"("Device Name"="x_calc") -> ("Truncated Data History"=w394:T12)  [unwired: 7 in, 3 out]
    n190 = Unbundle(w396) -> (w395:cluster{"Time Stamp":dbl, "Data Value":dbl}[])
    n191 = Unbundle(w394) -> (w393:cluster{"Time Stamp":dbl, "Data Value":dbl}[])
    n192 = for {
      tunnel: w395 -> [w417] mode=indexing
      tunnel: w393 -> [w416] mode=indexing
      tunnel: [w414] -> w378 mode=indexing
      tunnel: [w413] -> w371 mode=indexing
      tunnel: [w412] -> w372 mode=indexing
      n193 = Unbundle By Name(w417) -> ("Data Value"=w412:dbl)
      n194 = Unbundle By Name(w416) -> ("Data Value"=w413:dbl)
      n195 = Bundle By Name(cluster=cluster{"Time Stamp":dbl, "Data Value":dbl} {"Time Stamp"=0.0, "Data Value"=0.0}, "Data Value"=w412, "Time Stamp"=w413) -> (w414:cluster{"Time Stamp":dbl, "Data Value":dbl})
    }
    n196 = for {
      tunnel: string[] ["elevator", "rudder", "theta", "phi", "psi", "aileron", "d_elevator", "d_aileron", "d_rudder", "d_motor"] -> [w420] mode=indexing
      tunnel: [w419] -> w407 mode=indexing
      tunnel: [w418] -> _ mode=indexing
      n197 = call "Read Data Xfer.vi"("Device Name"=w420) -> ("Latest Value"=w419:dbl, "Truncated Data History"=w418:T12)  [unwired: 7 in, 2 out]
    }
    n198 = call "Read Data Xfer.vi"("Device Name"="altitude") -> ("Truncated Data History"=w391:T12)  [unwired: 7 in, 3 out]
    n199 = call "Read Data Xfer.vi"("Device Name"="u") -> ("Latest Value"=→"Airspeed (ft/s)":dbl)  [unwired: 7 in, 3 out]
    n200 = call "Read Data Xfer.vi"("Device Name"="phi") -> ("Truncated Data History"=w365:T12)  [unwired: 7 in, 3 out]
    n201 = call "Read Data Xfer.vi"("Device Name"="psi") -> ("Truncated Data History"=w361:T12)  [unwired: 7 in, 3 out]
    n202 = call "Read Data Xfer.vi"("Device Name"="phi") -> ("Truncated Data History"=w355:T12)  [unwired: 7 in, 3 out]
    n203 = call "Read Data Xfer.vi"("Device Name"="d_aileron") -> ("Truncated Data History"=w360:T12)  [unwired: 7 in, 3 out]
    n204 = Build Array(w391) -> (→"altitude":T1)
    n205 = Build Array(w365) -> (→"plot":T1)
    n206 = Build Array(w361, w355) -> (→"altitude 3":T1)
    n207 = Build Array(w360) -> (→"altitude 2":T1)
    n208 = Index Array(array=w407) -> (element #1=w406:dbl, element #2=w400:dbl, element #3=w380:dbl, element #4=w381:dbl, element #5=w386:dbl, element #6=w401:dbl, element #7=→"elevator":dbl, element #8=→"aileron":dbl, element #9=→"rudder":dbl, element #10=→"motor (BHP)":dbl)  [unwired: 10 in]
    "roll" <- w381
    "pitch" <- w380
    n209 = control-ref of="ground track"() -> (w379:refnum<vi>)
    n210 = Negate(x=w401) -> (-x=w405:dbl)
    n211 = call "format_heading.vi"("Heading (deg)"=w386) -> ("heading (formatted)"=→"Heading":T2)
    n212 = property class="XYGraph (strict)"(reference=w379, "Value"=w378) -> (reference out=w377:refnum<vi>)  [unwired: 1 in, 1 out]
    n213 = Negate(x=w381) -> (-x=w382:dbl)
    n214 = call "3d_aircraft.vi"("RH Aileron"=w405, "Elevator"=w406, "LH Aileron"=w401, "Rudder"=w400, "Heading (deg)"=w386, "Roll (deg)"=w381, "Pitch (deg)"=w380, "visual"="visual") -> ()  [unwired: 4 in]
    n215 = Bundle By Name(cluster=T11 {"X"=0.0, "Y"=0.0, "Z"=0.0} ("Control 1"), "X"=w380, "Y"=w382, "Z"=w386) -> (w384:T11)
    n216 = Array Max & Min(array=w371) -> (max value=w370:dbl, min value=w369:dbl)  [unwired: 2 out]
    n217 = Array Max & Min(array=w372) -> (max value=w368:dbl, min value=w367:dbl)  [unwired: 2 out]
    n218 = call "Attitude Control Write.vi"("pitch (x), roll (y), yaw (z)"=w384, "Attitude Control Handle In"=w385) -> ("Attitude Control Handle Out"=w383:T9)  [unwired: 8 in, 1 out]
    n219 = call "axis equal in labview.vi"("y min"=w367, "y max"=w368, "x min"=w369, "x max"=w370) -> ("yscale min"=w373:dbl, "yscale max"=w374:dbl, "xscale min"=w375:dbl, "xscale max"=w376:dbl)  [unwired: 4 in]
    n220 = property class="XYGraph (strict)"(reference=w377, "XScale.Maximum"=w376, "XScale.Minimum"=w375, "YScale.Maximum"=w374, "YScale.Minimum"=w373) -> ()  [unwired: 1 in, 2 out]
    n221 = Wait (ms)(milliseconds to wait=u32 20) -> ()  [unwired: 1 out]
    n222 = local read "stop"() -> (w411:bool)
  }
  n223 = call "Attitude Control Close.vi"("Attitude Control Handle"=w52) -> ()  [unwired: 10 in, 1 out]
